vi "COmpute encoder distance drive.vi"(8 "error in (no error)":errorcluster, 9 "Right Starting":dbl, 10 "Left Starting":dbl, 11 "Wanted Distance":dbl) -> (0 "error out":errorcluster, 1 "Right Drive":dbl, 2 "Left Drive":dbl, 3 "Done":bool)   [LabVIEW 2017]
uses:
  <vilib>/Rock Robotics/WPI/ThirdParty/Phoenix-LabVIEW/Motor Controller/Controls/CTRE_Phoenix_MotorControl_FeedbackDevice.ctl
  <vilib>/Rock Robotics/WPI/ThirdParty/Phoenix-LabVIEW/Motor Controller/Get/CTRE_Phoenix_MotorController_GetSelectedSensorData.vi
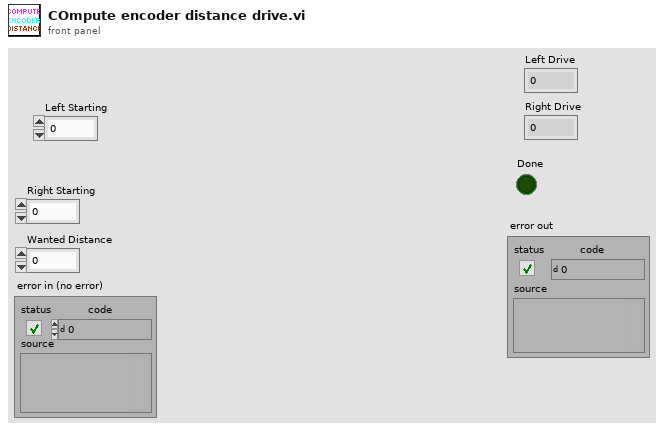
[diagram p1: front panel]
types:
  T1 = typedef "CTRE_Phoenix_MotorControl_FeedbackDevice.ctl" = i8
  T2 = typedef "WPI_MotorControlDeviceRef.ctl" = cluster{"DeviceStatus":errorcluster, "Type":T3, "PWM":cluster{"PWM Channel":T4, "DeadBand":T5}, "CAN":cluster{"Device Number":u8, "SetOutput VI Ref":variant, "GetOutput VI Ref":variant, "Enable VI Ref":variant, "Disable VI Ref":variant, "Data":variant}, "Invert":bool, "DIO PWM":cluster{"PWM \"Enable\" Channel":T4, "DIOChannel":T6, "PWM Rate":dbl}}
  T3 = typedef "WPI_MotorControlType.ctl" = enum16{"PWM", "CAN", "DIO PWM"}
  T4 = typedef "FPGA_DIOPWMChannel.ctl" = enum8{"PWM 0", "PWM 1", "PWM 2", "PWM 3", "PWM 4", "PWM 5", "PWM 6", "PWM 7", "PWM 8", "PWM 9", "PWM MXP 0", "PWM MXP 1", "PWM MXP 2", "PWM MXP 3", "PWM MXP 4", "PWM MXP 5", "PWM MXP 6", "PWM MXP 7", "PWM MXP 8", "PWM MXP 9", "Invalid"}
  T5 = typedef "WPI_PWMDeadband.ctl" = cluster{"Name":string, "maxPositivePwm":i32, "minPositivePwm":i32, "centerPwm":i32, "maxNegativePwm":i32, "minNegativePwm":i32, "angularRange":u16}
  T6 = typedef "FPGA_DIOChannel.ctl" = enum8{"DIO 0", "DIO 1", "DIO 2", "DIO 3", "DIO 4", "DIO 5", "DIO 6", "DIO 7", "DIO 8", "DIO 9", "DIO MXP 0", "DIO MXP 1", "DIO MXP 2", "DIO MXP 3", "DIO MXP 4", "DIO MXP 5", "DIO MXP 6", "DIO MXP 7", "DIO MXP 8", "DIO MXP 9", "DIO MXP 10", "DIO MXP 11", "DIO MXP 12", "DIO MXP 13", "DIO MXP 14", "DIO MXP 15", "SPI Port CS1", "SPI Port CS2", "SPI Port CS3", "SPI Port MISO", "SPI Port MOSI", "Invalid"}
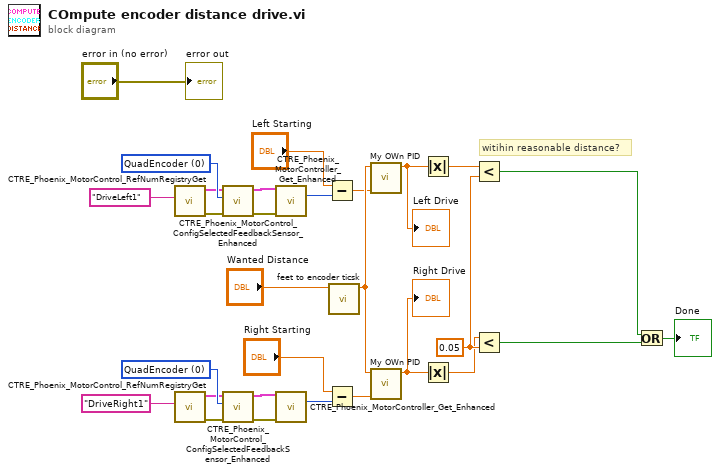
[diagram p0: block diagram]
diagram:
  w10 = T1 0 items=["None"=-1, "QuadEncoder"=0, "Analog"=2, "Tachometer"=4, "Pulse Width Encoded Position"=8, "Sensor Sum (S0 + S1)"=9, "Sensor Difference (D0 - D1)"=10, "Remote Source 0"=11, "Remote Source 1"=12, "Software Emulated"=15] ("Feedback Device")
  w13 = T1 0 items=["None"=-1, "QuadEncoder"=0, "Analog"=2, "Tachometer"=4, "Pulse Width Encoded Position"=8, "Sensor Sum (S0 + S1)"=9, "Sensor Difference (D0 - D1)"=10, "Remote Source 0"=11, "Remote Source 1"=12, "Software Emulated"=15] ("Feedback Device")
  w20 = 0.05
  # "witihin reasonable distance?"
  n1 = call <vilib>:"CTRE_Phoenix_MotorControl_RefNumRegistryGet.vi"("refnum name"="DriveLeft1") -> ("error out"=w6:errorcluster, "PhoenixMotorControlDevRef"=w9:T2)  [unwired: 9 in]
  n2 = call <vilib>:"CTRE_Phoenix_MotorControl_RefNumRegistryGet.vi"("refnum name"="DriveRight1") -> ("error out"=w15:errorcluster, "PhoenixMotorControlDevRef"=w12:T2)  [unwired: 9 in]
  n3 = call <vilib>:"CTRE_Phoenix_MotorControl_ConfigSelectedFeedbackSensor_Enhanced.vi"("error in (no error)"=w6, "Feedback Device"=w10, "PhoenixMotorControlDevRef"=w9) -> ("error out"=w7:errorcluster, "PhoenixMotorControlDevRef"=w8:T2)  [unwired: 7 in]
  n4 = call <vilib>:"CTRE_Phoenix_MotorControl_ConfigSelectedFeedbackSensor_Enhanced.vi"("error in (no error)"=w15, "Feedback Device"=w13, "PhoenixMotorControlDevRef"=w12) -> ("error out"=w14:errorcluster, "PhoenixMotorControlDevRef"=w11:T2)  [unwired: 7 in]
  n5 = call-poly <vilib>:"CTRE_Phoenix_MotorController_Get_Enhanced.vi"("PhoenixMotorControlDevRef"=w8, "error in"=w7) -> ("Position (Raw Sensor Units)"=w24:i32)  [unwired: 10 in, 3 out]
  n6 = call-poly <vilib>:"CTRE_Phoenix_MotorController_Get_Enhanced.vi"("PhoenixMotorControlDevRef"=w11, "error in"=w14) -> ("Position (Raw Sensor Units)"=w23:i32)  [unwired: 10 in, 3 out]
  n7 = Subtract(x="Left Starting", y=w24) -> (x-y=w22:dbl)
  n8 = Subtract(x="Right Starting", y=w23) -> (x-y=w21:dbl)
  n9 = call "feet to encoder ticsk.vi"("Distance in feet wanted"="Wanted Distance") -> ("Encoder Ticks"=w28:dbl)  [unwired: 10 in]
  n10 = call "My OWn PID.vi"("Current Input"=w22, "Wanted End"=w28) -> ("Output"=w5:dbl)  [unwired: 9 in]
  "Left Drive" <- w5
  n11 = call "My OWn PID.vi"("Current Input"=w21, "Wanted End"=w28) -> ("Output"=w4:dbl)  [unwired: 9 in]
  "Right Drive" <- w4
  n12 = Absolute Value(x=w5) -> (abs(x)=w16:dbl)
  n13 = Absolute Value(x=w4) -> (abs(x)=w17:dbl)
  n14 = Less?(x=w16, y=w20) -> (x < y?=w19:bool)
  n15 = Less?(x=w17, y=w20) -> (x < y?=w18:bool)
  n16 = Or(x=w19, y=w18) -> (x .or. y?=→"Done":bool)
  "error out" <- "error in (no error)"
